vi "远程本地判断.vi"(1 "toHMI本地":bool, 2 "toHMI远程":bool) -> (0 "远程/本地":enum16{"零位", "本地", "远方"}(ring))   [LabVIEW 2015]
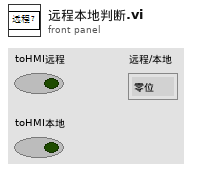
[diagram p1: front panel]
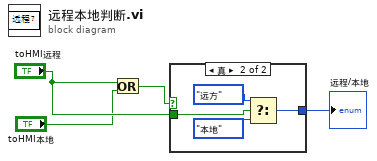
[diagram p0: block diagram]
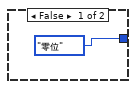
[diagram p2: hidden frame]
diagram:
  n1 = Or(x="toHMI远程", y="toHMI本地") -> (x .or. y?=w2:bool)
  n2 = case shown="真" w2 {
    tunnel: [enum16{"零位", "本地", "远方"}."零位" ("远程/本地") w6] -> w3
    tunnel: "toHMI远程" -> [_ w7]
    frame False {
    }
    frame True {
      n3 = Select(t=enum16{"零位", "本地", "远方"}."远方" ("远程/本地"), s=w7, f=enum16{"零位", "本地", "远方"}."本地" ("远程/本地")) -> (s? t:f=w6:enum16{"零位", "本地", "远方"})
    }
  }
  "远程/本地" <- w3
